vi "Get_PAQpointers.vi"(8 "error in (no error)":errorcluster, 11 "FAMM in":refnum<class "FAMM.lvclass">) -> (0 "error out":errorcluster, 2 "PAQpointers":i32[](array[numeric]), 3 "FAMM out":refnum<class "FAMM.lvclass">)   [LabVIEW 2020, in "FAMM.lvclass"]
doc: "Read all PAQ pointers"
uses:
  FAMM.lvclass
  FAMM.lvclass/FAMM.ctl
  PAQ-memory.lvclass/PAQ-memory.ctl
  PAQ-memory.lvclass
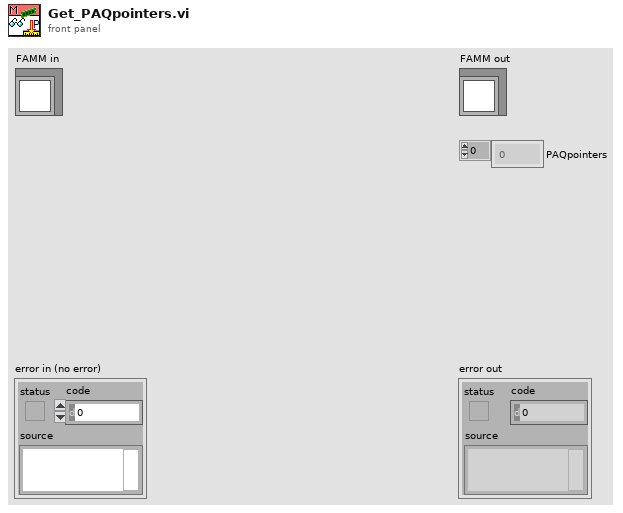
[diagram p1: front panel]
types:
  T1 = typedef "FAMM.lvclass/FAMM-attributes.ctl" = cluster{"FAMM_PAQ_Layers":i32, "FAMM_PAQ_resolution":dbl, "PAQ_TAGs":string[], "WAQ_TAGs":string[], "EAQ_TAGs":string[], "All_TAGs":string[], "PAQtagProps":T2[], "WAQtagProps":T2[], "EAQtagProps":T2[], "DBAL_class":refnum<data-value>, "PAQ_memory":refnum<data-value>[], "PAQupdates":timestamp[], "FAMM_Size":cluster{"other":i32, "1day":i32, "1week":i32}, "DatabaseFileExtention":string, "DatabaseSaveRate":dbl, "Database_path":path}
  T2 = typedef "typedef_com_TagProp.ctl" = cluster{"Description":string, "EngUnits":string, "RangeH":dbl, "RangeL":dbl, "Resolution":i32, "Obsolete":bool, "ChangeDate":timestamp, "ChangeSource":string, "ChangeReason":string, "TagFunc":u32}
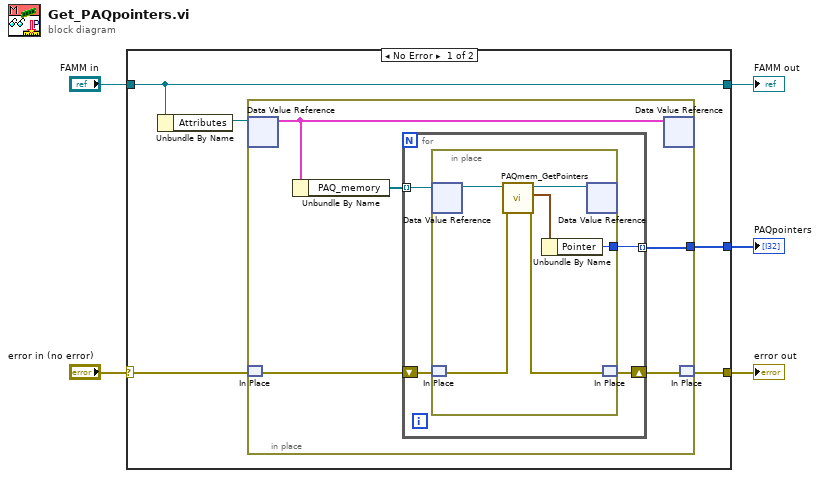
[diagram p0: block diagram]
diagram:
  n1 = case shown="No Error" "error in (no error)" {
    selector: "error in (no error)" -> [w9 w26]
    tunnel: [w8 w26] -> w4
    tunnel: [w7 w27] -> w2
    tunnel: "FAMM in" -> [w7 w27]
    tunnel: [w10 _] -> w1
    frame No Error {
      n2 = Unbundle By Name(w7) -> ("Attributes"=w6:refnum<data-value>)
      n3 = in-place {
        in-place-border: [w12] -> w10
        n4 = in-place-dvr #1(w6) -> (w15:T1)  [unwired: 1 out]
        n5 = in-place-match #2(w9) -> (w13:errorcluster)
        n6 = Unbundle By Name(w15) -> ("PAQ_memory"=w14:refnum<data-value>[])
        n7 = for {
          tunnel: w14 -> [w19] mode=indexing
          shift-right: [w17] -> w11
          shift-left: w13 -> [w16]
          tunnel: [w18] -> w12 mode=indexing
          n8 = in-place {
            in-place-border: [w21] -> w18
            n9 = in-place-dvr #3(w19) -> (w25:refnum<class "PAQ-memory.lvclass">)  [unwired: 1 out]
            n10 = in-place-match #4(w16) -> (w20:errorcluster)
            n11 = call "PAQmem_GetPointers.vi"("error in (no error)"=w20, "PAQ-memory in"=w25) -> ("error out"=w23:errorcluster, "Pointers"=w22:cluster{"Pointer":i32, "Carry":i32}, "PAQ-memory out"=w24:refnum<class "PAQ-memory.lvclass">)  [unwired: 7 in]
            n12 = Unbundle By Name(w22) -> ("Pointer"=w21:i32)
            n13 = in-place-dvr #3(w24) -> ()  [unwired: 2 out]
            n14 = in-place-match #4(w23) -> (w17:errorcluster)
          }
        }
        n15 = in-place-dvr #1(w15) -> ()  [unwired: 2 out]
        n16 = in-place-match #2(w11) -> (w8:errorcluster)
      }
    }
    frame Error {
    }
  }
  "error out" <- w4
  "FAMM out" <- w2
  "PAQpointers" <- w1
